vi "_config-pic.vi"() -> ()   [LabVIEW 2019]
panel:
  in  "Tab Control":enum32{"DL950", "BP4610", "DSP1500", "ai", "ao"}(tab)
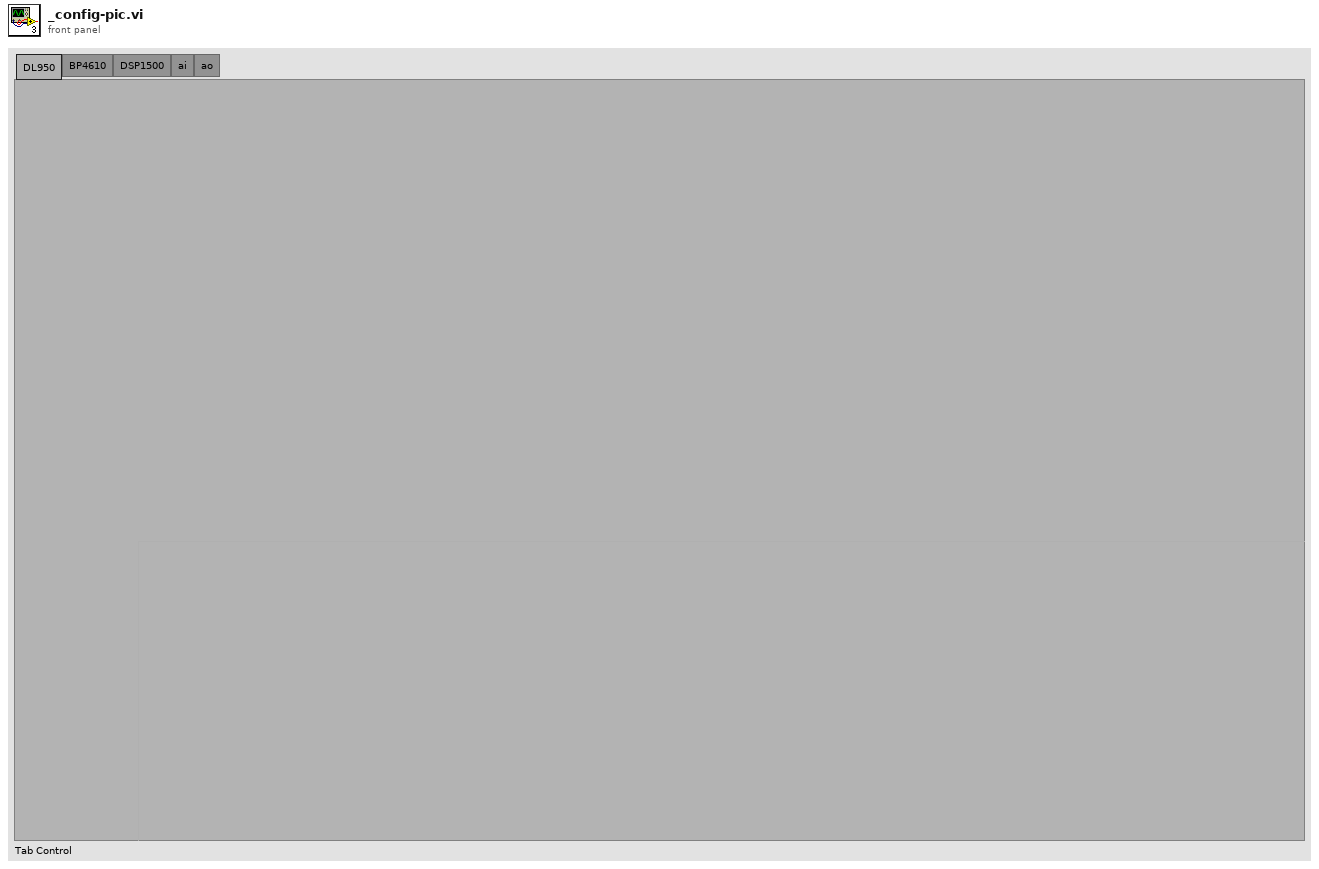
[diagram p1: front panel]
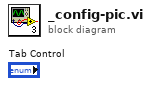
[diagram p0: block diagram]
diagram:
